vi "Receive.vi"(6 "Timeout":T2={"mode"=enum."Relative", "deadline (ms)"=30000}, 8 "error in (no error)":errorcluster, 9 "request id":u32, 10 "session in":refnum<class "Session.lvclass">, 11 "NI_SFTP.lvlib:fstatvfs_openssh.com.lvclass":refnum<class "fstatvfs_openssh.com.lvclass">) -> (0 "error out":errorcluster, 1 "statistics":T1 {"f_flag" format="%x"; "f_fsid" format="%x"}, 2 "session out":refnum<class "Session.lvclass">, 3 "NI_SFTP.lvlib:fstatvfs_openssh.com.lvclass 2":refnum<class "fstatvfs_openssh.com.lvclass">)   [LabVIEW 2020, in "NI_SFTP.lvlib" / "fstatvfs_openssh.com.lvclass"]
uses:
  <vilib>/net/SFTP/API/Support/Command/fstatvfs_openssh.com/fstatvfs_openssh.com.lvclass
  <vilib>/net/SFTP/Session/Session.lvclass
  <vilib>/Utility/Deadline/Deadline.ctl
  <vilib>/Utility/Deadline/Mode.ctl
  <vilib>/net/SFTP/API/Support/statvfs info.ctl
  <vilib>/Utility/error.llb/Error Cluster From Error Code.vi
  <vilib>/ErrorRing/Error Ring.xnode
  <vilib>/net/SFTP/API/Support/Command/SSH_FXP_EXTENDED/SSH_FXP_EXTENDED.lvclass
  <vilib>/net/SFTP/NI_SFTP.lvlib
  <vilib>/Utility/Deadline/NI_Deadline.lvlib
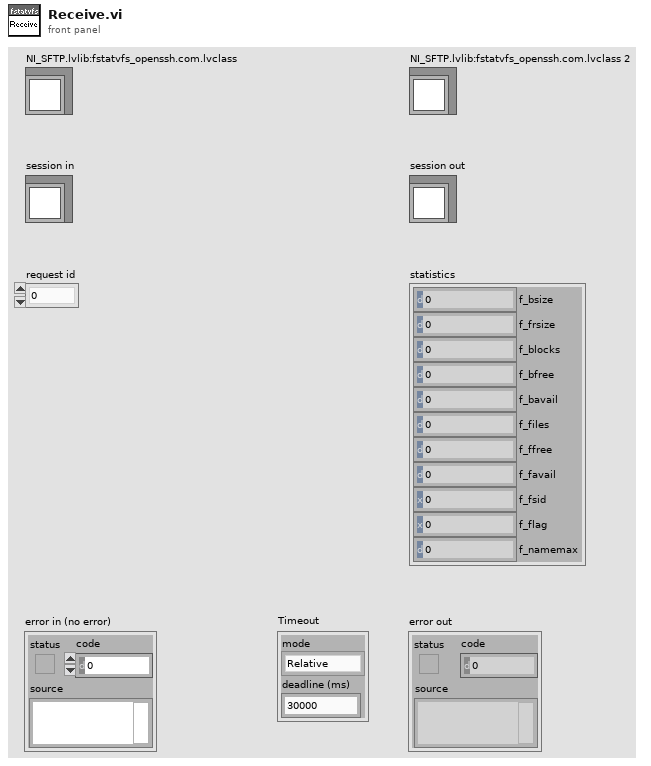
[diagram p1: front panel]
types:
  T1 = typedef "NI_SFTP.lvlib/statvfs info.ctl" = cluster{"f_bsize":u64, "f_frsize":u64, "f_blocks":u64, "f_bfree":u64, "f_bavail":u64, "f_files":u64, "f_ffree":u64, "f_favail":u64, "f_fsid":u64, "f_flag":u64, "f_namemax":u64}
  T2 = typedef "NI_Deadline.lvlib/Deadline.ctl" = cluster{"mode":T3, "deadline (ms)":u32}
  T3 = typedef "NI_Deadline.lvlib/Mode.ctl" = enum16{"Relative", "Use deadline", "Wait forever", "Nonblocking", "N/A"}
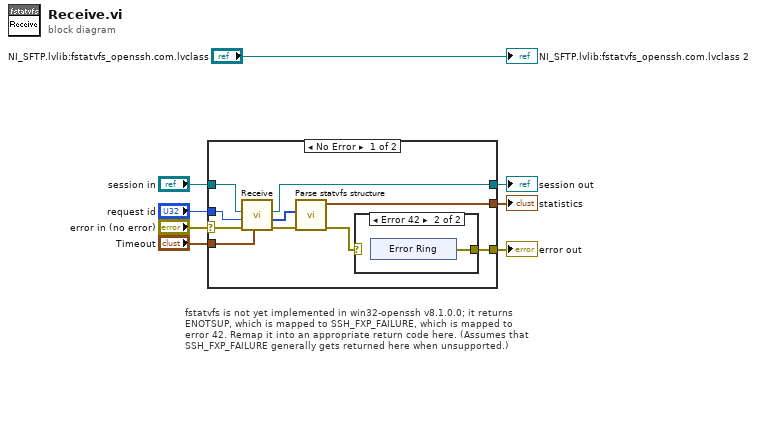
[diagram p0: block diagram]
diagram:
  # "fstatvfs is not yet implemented in win32-openssh v8.1.0.0; it returns ENOTSUP, which is mapped to SSH_FXP_FAILURE, which is mapped to error 42. Remap it into an appropriate return code here. (Assumes that SSH_FXP_FAILURE generally gets returned here when unsupported.)"
  n1 = case shown="No Error" "error in (no error)" {
    selector: "error in (no error)" -> [w18 w26]
    tunnel: "request id" -> [w10 _]
    tunnel: "session in" -> [w11 w25]
    tunnel: [w12 w25] -> w6
    tunnel: [w13 w26] -> w5
    tunnel: "Timeout" -> [w17 _]
    tunnel: [w15 _] -> w2
    frame No Error {
      n2 = call <vilib>:"Receive.vi"("deadline"=w17, "error in (no error)"=w18, "request id"=w10, "session in"=w11) -> ("error out"=w16:errorcluster, "payload"=w9:u8[], "session out"=w12:refnum<class "Session.lvclass">)  [unwired: 4 in, 1 out]
      n3 = call <vilib>:"Parse statvfs structure.vi"("error in (no error)"=w16, "payload"=w9) -> ("error out"=w14:errorcluster, "statvfs"=w15:T1)  [unwired: 8 in]
      n4 = case shown="Error 42" w14 {
        selector: w14 -> [w19 _]
        tunnel: [w19 w20] -> w13
        frame #0 {
        }
        frame #1 {
          n5 = xnode "Error Ring"() -> ("error out"=w20:errorcluster)
        }
      }
    }
    frame Error {
    }
  }
  "error out" <- w5
  "session out" <- w6
  "statistics" <- w2
  "NI_SFTP.lvlib:fstatvfs_openssh.com.lvclass 2" <- "NI_SFTP.lvlib:fstatvfs_openssh.com.lvclass"
